vi "Filter for interesting controls.vi"(8 "Error in":errorcluster, 10 "All FP control references":refnum<vi>[](array[refnum]), 11 "Interesting control names":string[](array[string])) -> (0 "Error out":errorcluster, 3 "Matched controls":refnum<vi>[](array[refnum]))   [LabVIEW 2019, in "LSS.lvlib"]
doc: "Uses the list of controls that are used in the rules and finds their associated references.\n\n<b>Inputs:</b>\n<b>Interesting control names</b> - List of controls that have defined rules.\n<b>All FP control references</b> - List of controls references to search through to find the relevent controls.\n<b>Error In</b> - Standard Error In terminal.\n\n<b>Outputs:</b>\n<b>Matched controls</b> - Controls that have defined rules. The property control engine must register for their value change events.\n<b>Error Out</b> - Standard Error out terminal."
uses:
  LSS.lvlib
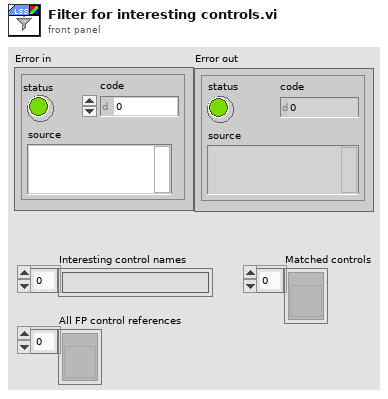
[diagram p1: front panel]
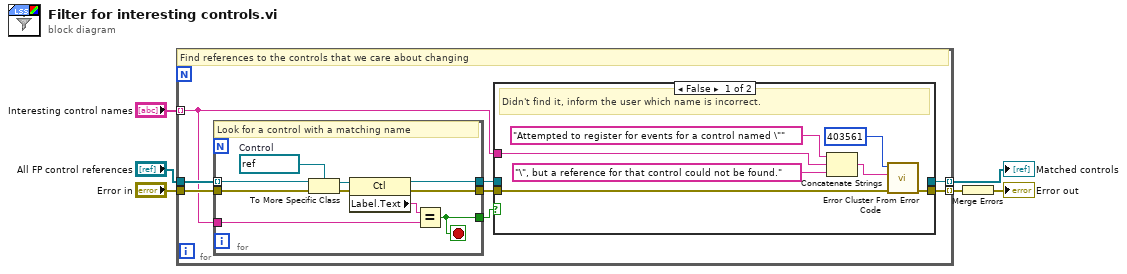
[diagram p0: block diagram]
diagram:
  n1 = for {
    tunnel: "All FP control references" -> [w14]
    tunnel: "Interesting control names" -> [w8] mode=indexing
    tunnel: [w11] -> w5 mode=indexing
    tunnel: "Error in" -> [w13]
    tunnel: [w7] -> w2 mode=indexing
    # "Find references to the controls that we care about changing"
    n2 = for {
      tunnel: w8 -> [w32]
      tunnel: [w29] -> w12
      tunnel: w13 -> [w25]
      tunnel: w14 -> [w33] mode=indexing
      tunnel: [w30] -> w10
      tunnel: [w26] -> w9
      stop <- w29 stop-if-true
      w27 = refnum<vi> refnum  # Control
      # "Look for a control with a matching name"
      n3 = To More Specific Class(target class=w27, reference=w33, error in=w25) -> (specific class reference=w28:refnum<vi>, error out=w24:errorcluster)
      n4 = property class="Ctl"(reference=w28, error in=w24) -> (reference out=w30:refnum<vi>, error out=w26:errorcluster, "Label.Text"=w31:string)
      n5 = Equal?(x=w31, y=w32) -> (x = y?=w29:bool)
    }
    n6 = case shown="False" w12 {
      tunnel: [_ w23] -> w11
      tunnel: w10 -> [_ w23]
      tunnel: w9 -> [w21 w22]
      tunnel: w8 -> [w17 _]
      tunnel: [w15 w22] -> w7
      frame False {
        # "Didn't find it, inform the user which name is incorrect."
        n7 = Concatenate Strings("Attempted to register for events for a control named \"" ("error message (\"\")"), w17, "\", but a reference for that control could not be found." ("string")) -> (w18:string)
        n8 = call <vilib>:"Error Cluster From Error Code.vi"("error in (no error)"=w21, "error message (\"\")"=w18, "error code (0)"=403561) -> ("error out"=w15:errorcluster)  [unwired: 6 in]
      }
      frame True {
        # "Found the control, move along"
      }
    }
  }
  "Matched controls" <- w5
  n9 = Merge Errors(w2) -> (→"Error out":errorcluster)
